vi "euler_diff.vi"(1 "dt":dbl=0.02, 2 "Input":dbl) -> (0 "Output":dbl)   [LabVIEW 2021]
doc: "Finite difference method + low pass filter"
uses:
  <vilib>/Analysis/3filter.llb/Filter Passband Type.ctl
  <vilib>/ptbypt/NI_PtbyPt.lvlib
  <vilib>/Analysis/NI_AALBase.lvlib
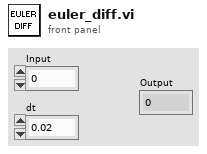
[diagram p1: front panel]
types:
  T1 = typedef "NI_AALBase.lvlib/Filter Passband Type.ctl" = enum32{"Lowpass", "Highpass", "Bandpass", "Bandstop"}
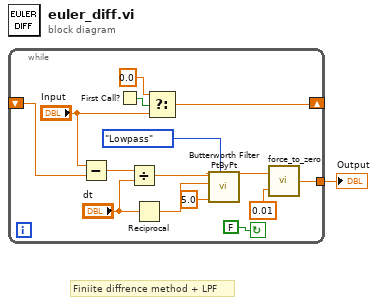
[diagram p0: block diagram]
diagram:
  # "Finiite diffrence method + LPF"
  n1 = while {
    shift-right: [w14] -> _
    shift-left: _ -> [w12]
    tunnel: [w4] -> w1
    stop <- FALSE continue-if-true
    n2 = Subtract(x="Input", y=w12) -> (x-y=w10:dbl)
    n3 = First Call?() -> (First Call?: T/F=w15:bool)
    n4 = Divide(x=w10, y="dt") -> (x/y=w9:dbl)
    n5 = Reciprocal(x="dt") -> (1/x=w7:dbl)
    n6 = Select(t=0.0, s=w15, f="Input") -> (s? t:f=w14:dbl)
    n7 = call <vilib>:"Butterworth Filter PtByPt.vi"("filter type"=Filter_Passband_Type."Lowpass", "low cutoff freq: fl"=5.0, "sampling freq: fs"=w7, "x"=w9) -> ("Filtered x"=w3:dbl)  [unwired: 5 in, 1 out]
    n8 = call "force_to_zero.vi"("Epsilon"=0.01, "Input"=w3) -> ("Output"=w4:dbl)
  }
  "Output" <- w1
